vi "HRNorm.vi"(6 "Target Heart Rate":dbl, 9 "HR_max":dbl, 10 "HR_rest":dbl, 11 "x1":u32) -> (1 "eHR":dbl, 2 "x1_norm":dbl, 3 "x1_ref_norm":dbl)   [LabVIEW 2013]
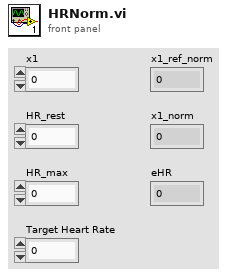
[diagram p1: front panel]
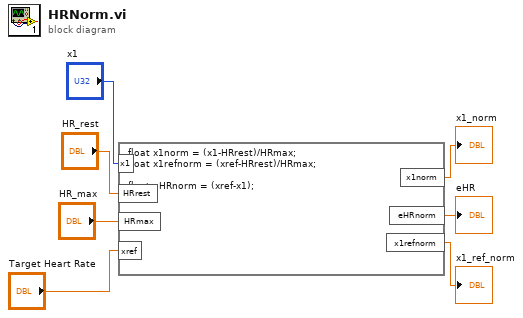
[diagram p0: block diagram]
diagram:
  n1 = formula code="float x1norm = (x1-HRrest)/HRmax;\nfloat x1refnorm = (xref-HRrest)/HRmax;\n\nfloat eHRnorm = (xref-x1);"("x1"="x1", "HRrest"="HR_rest", "HRmax"="HR_max", "xref"="Target Heart Rate") -> ("x1norm"=→"x1_norm":dbl, "eHRnorm"=→"eHR":dbl, "x1refnorm"=→"x1_ref_norm":dbl)
